vi "Do_GetObjectConfiguration.vi"(8 "Error In":errorcluster, 10 "ConfigSource":refnum<class "IApplicationConfiguration.lvclass">, 11 "ApplicationIn":refnum<class "Application.lvclass">) -> (0 "Error Out":errorcluster, 2 "ConfigSourceOut":refnum<class "IApplicationConfiguration.lvclass">, 3 "ApplicationOut":refnum<class "Application.lvclass">)   [LabVIEW 2021, in "Application.lvclass"]
uses:
  Application.lvclass
  Interface_TAF_IApplicationConfiguration/IApplicationConfiguration/IApplicationConfiguration.lvclass
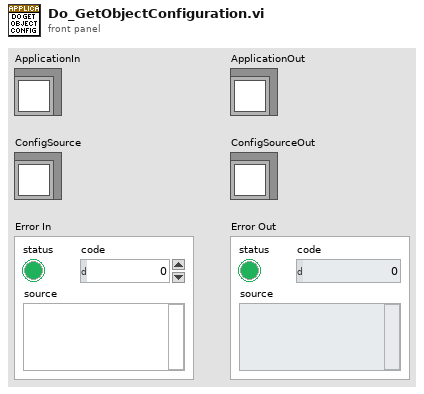
[diagram p1: front panel]
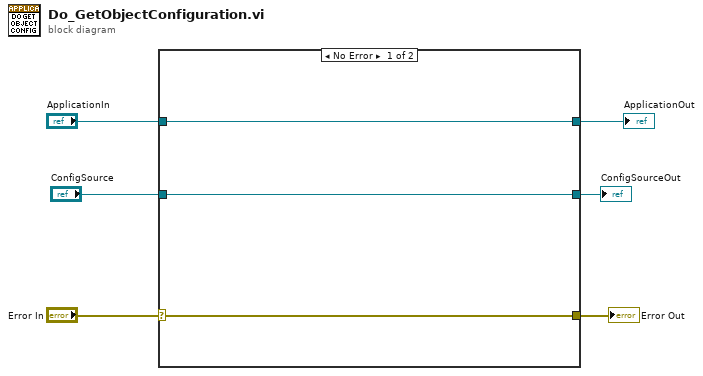
[diagram p0: block diagram]
diagram:
  n1 = case shown="No Error" "Error In" {
    selector: "Error In" -> [w8 w12]
    tunnel: [w8 w12] -> w5
    tunnel: "ConfigSource" -> [w7 w10]
    tunnel: [w9 w11] -> w2
    tunnel: "ApplicationIn" -> [w9 w11]
    tunnel: [w7 w10] -> w1
    frame No Error {
    }
    frame Error {
    }
  }
  "Error Out" <- w5
  "ApplicationOut" <- w2
  "ConfigSourceOut" <- w1
